vi "Change Buttons Position.vi"(8 "error in (no error)":errorcluster, 11 "MainUI in":refnum<class "UI_Top_Customer.lvclass">) -> (0 "error out":errorcluster, 3 "MainUI out":refnum<class "UI_Top_Customer.lvclass">)   [LabVIEW 2021, in "UI_Top_Customer.lvclass"]
uses:
  UI_Top_Customer.lvclass
  C:/Program Files (x86)/National Instruments/LabVIEW 2021/user.lib/John_Lib/AbstractActorTemplate/AbstractActorTemplate/UIActorTop.lvclass
  <vilib>/Utility/miscctls.llb/LVRectTypeDef.ctl
  UI_Top_Customer.lvclass/UI_Top_Customer.ctl
panel:
  out "Front Panel Window:Panel Bounds":T1
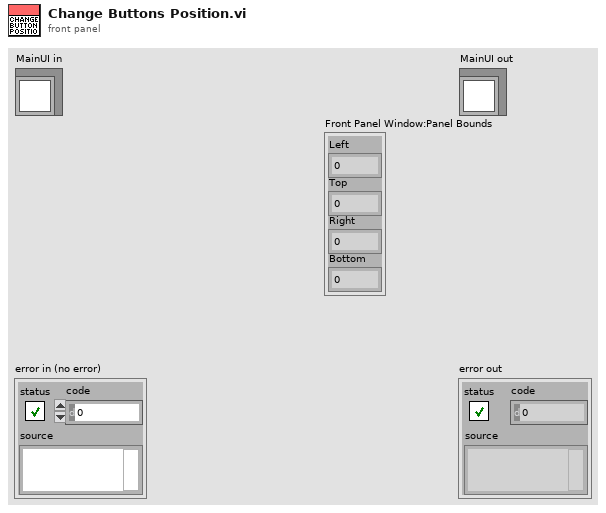
[diagram p1: front panel]
types:
  T1 = typedef "LVRectTypeDef.ctl" = cluster{"Left":i16, "Top":i16, "Right":i16, "Bottom":i16}
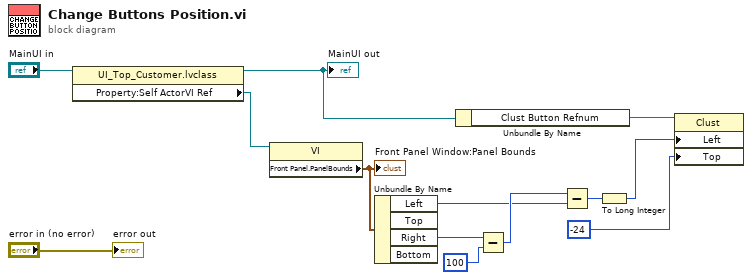
[diagram p0: block diagram]
diagram:
  n1 = property class="UI_Top_Customer.lvclass"(reference="MainUI in") -> (reference out=w10:refnum<class "UI_Top_Customer.lvclass">, "Property:Self ActorVI Ref"=w12:refnum<vi>)  [unwired: 1 in, 1 out]
  "MainUI out" <- w10
  n2 = property class="VI"(reference=w12) -> ("Front Panel.PanelBounds"=w4:T1)  [unwired: 1 in, 2 out]
  "Front Panel Window:Panel Bounds" <- w4
  n3 = Unbundle By Name(w4) -> ("Left"=w5:i16, "Right"=w6:i16)  [unwired: 2 out]
  n4 = Unbundle By Name(w10) -> ("Clust Button Refnum"=w9:refnum<vi>)
  n5 = Subtract(x=w6, y=i16 100) -> (x-y=w8:i16)
  n6 = Subtract(x=w8, y=w5) -> (x-y=w2:i16)
  n7 = To Long Integer(number=w2) -> (32bit integer=w1:i32)
  n8 = property class="Clust"(reference=w9, "Left"=w1, "Top"=-24 ("Position:Top")) -> ()  [unwired: 1 in, 2 out]
  "error out" <- "error in (no error)"
